vi "Main.vi"() -> ()   [LabVIEW 2015, in "Stock.lvlib"]
doc: "This template is based off of the Queued Message Handler design pattern and the Queued Message Handler project template that ships with LabVIEW.\n\nThe main difference is that the queue is private to this module and communication between modules is performed via Broadcast and Request events.\n\nRequest events are wrapped in public API methods and are handled in the Event Handling Loop (EHL) of this VI. Any module can register for Broadcast events sent by this module. The EHL generates messages based on user interface actions.\n\nThe Message Handling Loop (MHL) processes messages generated by the EHL, or by other messages. The messages are string values, so new messages can be added easily to the Message Cases case structure in the MHL. Each message cluster can also provide an optional value for Message Data, which is a variant that can be converted to whatever message-specific data is required.\n_____\nBased on Delacor QMH Project Template 4.2.1.64."
uses:
  Stock.lvlib
  <vilib>/Delacor/Delacor QMH/Libraries/Module Admin_class/Delacor_lib_QMH_Module Admin.lvclass
  Module Data--cluster.ctl
  Products.ctl
  <vilib>/Delacor/Delacor QMH/Libraries/Message Queue_class/Delacor_lib_QMH_Message Queue.lvclass/Delacor_lib_QMH_Message Queue.ctl
  Stop Argument--cluster.ctl
  <vilib>/Delacor/Delacor QMH/Libraries/Module Admin_class/Delacor_lib_QMH_Module Admin.lvclass/Delacor_lib_QMH_Module Admin.ctl
  In Stock and Price Argument--cluster.ctl
  In Stock and Price (Reply Payload)--cluster.ctl
  Reduce Stock Level Argument--cluster.ctl
  Reduce Stock Level (Reply Payload)--cluster.ctl
  <vilib>/Utility/miscctls.llb/LVPointTypeDef.ctl
  <vilib>/Delacor/Delacor QMH/Libraries/Message Queue_class/Delacor_lib_QMH_Enqueue Message (Single).vi
  <vilib>/Delacor/Delacor QMH/Libraries/Module Admin_class/Delacor_lib_QMH_Get External Launch.vi
  <vilib>/Utility/error.llb/Error Cluster From Error Code.vi
  <vilib>/ErrorRing/Error Ring.xnode
  <vilib>/Delacor/Delacor QMH/Libraries/Message Queue_class/Delacor_lib_QMH_Message Queue.lvclass
panel:
  out "Stock Levels":T1(array[cluster]) {"Price" format="£%.2f"; "Stock Level" scale=0.0..58.0}
  in  "Simulate MHL Error":bool
  in  "Simulate EHL Error":bool
  out "error out":errorcluster
  in  "Module Admin":refnum<class "Delacor_lib_QMH_Module Admin.lvclass">
  out "Status":string
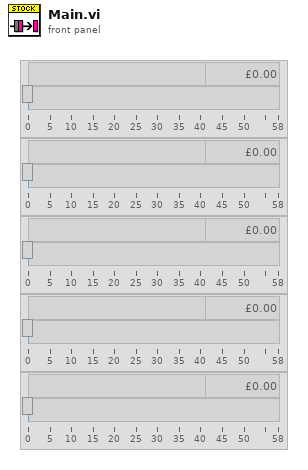
[diagram p1: front panel]
types:
  T1 = cluster{"Name":string, "Price":dbl, "Stock Level":dbl}[]
  T2 = typedef "Stock.lvlib/Request Events--cluster.ctl" = cluster{"Stop Module":refnum<user-event>, "Show Panel":refnum<user-event>, "Hide Panel":refnum<user-event>, "Get Module Execution Status":refnum<user-event>, "Show Diagram":refnum<user-event>, "In Stock and Price":refnum<user-event>, "Reduce Stock Level":refnum<user-event>}
  T3 = typedef "Stock.lvlib/Module Data--cluster.ctl" = cluster{"Status":string, "Stock":T4[], "Stock File Path":path}
  T4 = typedef "Stock.lvlib/Products.ctl" = cluster{"Name":string, "Price (pence/cents)":u32, "Stock Level":u32}
  T5 = enum32{"invalid lock state", "Not Locked", "Locked (No Password)", "Password-protected"}
  T6 = typedef "Stock.lvlib/Stop Argument--cluster.ctl" = cluster{"Origin":string, "Exit via Stop Module Req?":bool, "Wait for Module to stop?":bool}
  T7 = typedef "Stock.lvlib/In Stock and Price Argument--cluster.ctl" = cluster{"Stock Item":u32, "Wait Notifier":refnum<notifier>, "wait for reply":bool}
  T8 = typedef "Stock.lvlib/Reduce Stock Level Argument--cluster.ctl" = cluster{"Product":i32, "Wait Notifier":refnum<notifier>, "wait for reply":bool}
  T9 = typedef "LVPointTypeDef.ctl" = cluster{"Horizontal":i16, "Vertical":i16}
  T10 = typedef "Stock.lvlib/In Stock and Price (Reply Payload)--cluster.ctl" = cluster{"In Stock?":bool, "Price (Pence)":u32, "In Stock and Price_error":errorcluster}
  T11 = typedef "Stock.lvlib/Reduce Stock Level (Reply Payload)--cluster.ctl" = cluster{"Sucessful?":bool, "Reduce Stock Level_error":errorcluster}
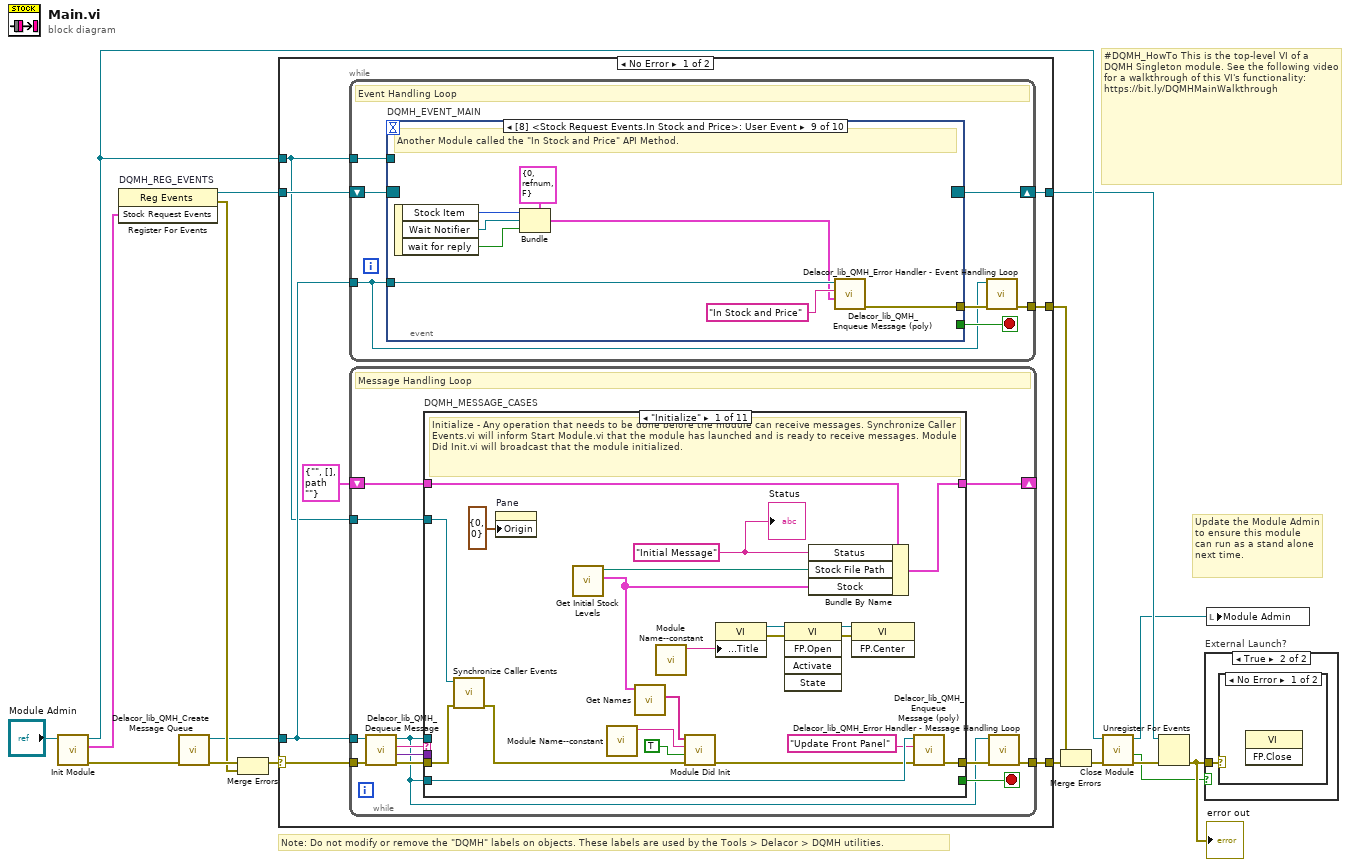
[diagram p0: block diagram]
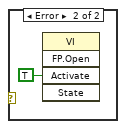
[diagram p3: hidden frame]
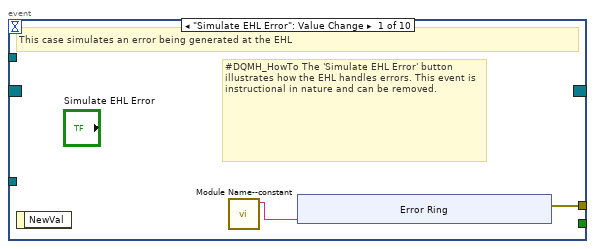
[diagram p4: hidden frame]
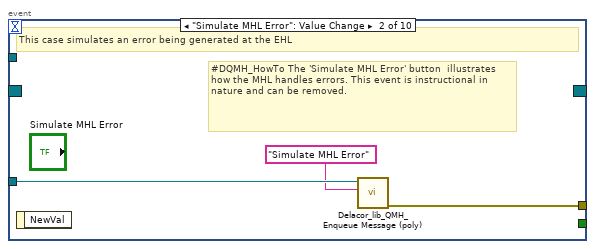
[diagram p5: hidden frame]
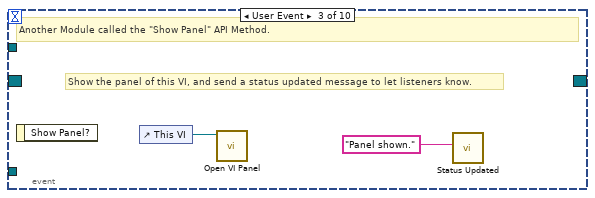
[diagram p6: hidden frame]
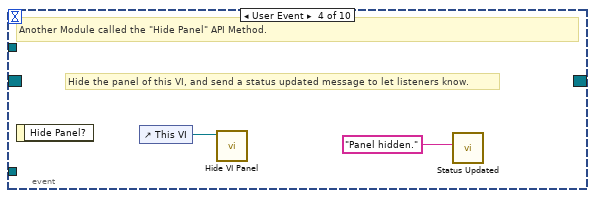
[diagram p7: hidden frame]
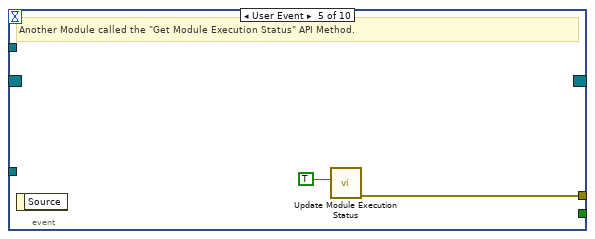
[diagram p8: hidden frame]
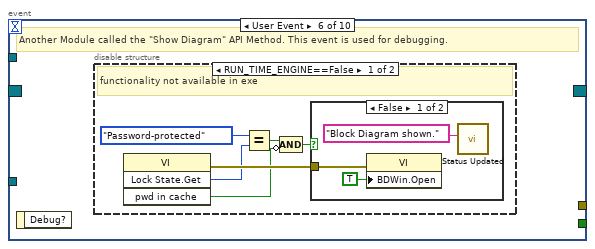
[diagram p9: hidden frame]
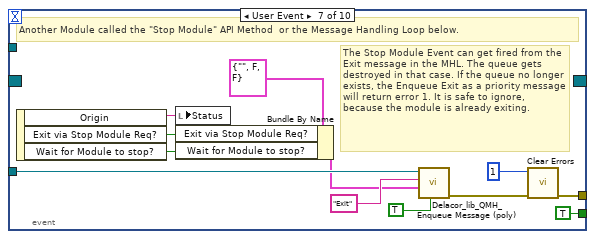
[diagram p12: hidden frame]
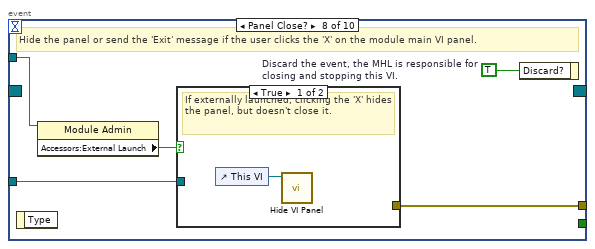
[diagram p13: hidden frame]
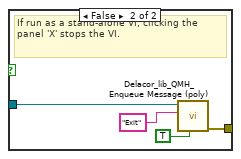
[diagram p14: hidden frame]
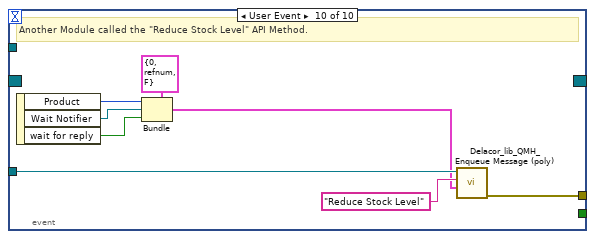
[diagram p15: hidden frame]
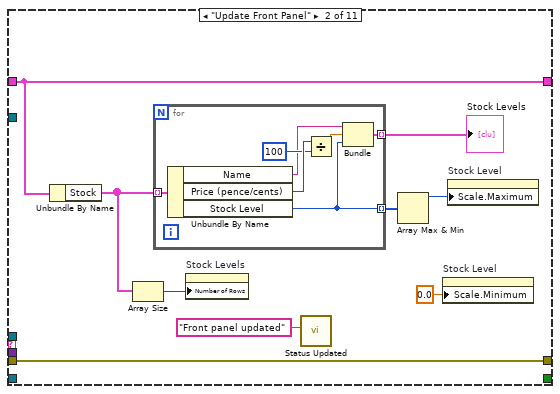
[diagram p16: hidden frame]
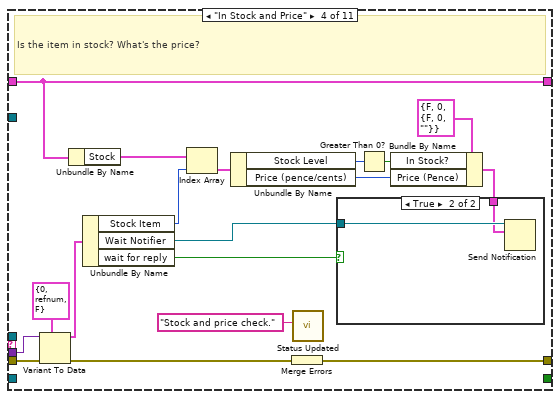
[diagram p18: hidden frame]
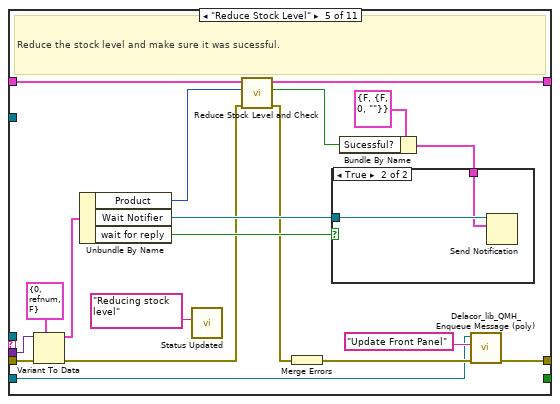
[diagram p20: hidden frame]
diagram:
  # "#DQMH_HowTo This is the top-level VI of a DQMH Singleton module. See the following video for a walkthrough of this VI's functionality: https://bit.ly/DQMHMainWalkthrough"
  # "Note: Do not modify or remove the \"DQMH\" labels on objects. These labels are used by the Tools > Delacor > DQMH utilities."
  # "Update the Module Admin to ensure this module can run as a stand alone next time."
  n1 = call "Init Module.vi"("Singleton Module Admin in"="Module Admin") -> ("error out"=w16:errorcluster, "Stock Request Events"=w5:T2, "Singleton Module Admin out"=w8:refnum<class "Delacor_lib_QMH_Module Admin.lvclass">)  [unwired: 8 in]
  n2 = register-events "DQMH_REG_EVENTS"(w5) -> (reference out=w6:refnum<event-registration>, error out=w9:errorcluster)  [unwired: 2 in]
  n3 = call <vilib>:"Delacor_lib_QMH_Create Message Queue.vi"("error in (no error)"=w16) -> ("error out"=w11:errorcluster, "Message Queue"=w4:refnum<class "Delacor_lib_QMH_Message Queue.lvclass">)  [unwired: 9 in]
  n4 = Merge Errors(w11, w9) -> (w10:errorcluster)
  n5 = case shown="No Error" w10 {
    selector: w10 -> [w23 w259]
    tunnel: [w25 w259] -> w17
    tunnel: [w22 w256] -> w7
    tunnel: w6 -> [w20 w256]
    tunnel: w4 -> [w19 _]
    tunnel: [w24 _] -> w14
    tunnel: w8 -> [w18 w252]
    frame No Error {
      n6 = while {
        tunnel: w19 -> [w26]
        shift-right: [w29] -> w22
        shift-left: w20 -> [w30]
        tunnel: [w31] -> w24
        tunnel: w18 -> [w27]
        stop <- w28 stop-if-true
        # "Event Handling Loop"
        n7 = event "DQMH_EVENT_MAIN" shown="[8] <Stock Request Events.In Stock and Price>: User Event" {
          selector: w30 -> [_ _ _ _ _ _ _ _ _ _]
          dyn-events: [_ _ _ _ _ _ _ _ _ _] -> w29
          timeout: _ -> [_ _ _ _ _ _ _ _ _ _]
          tunnel: [_ _ _ _ _ _ TRUE ("Discard?") _ _ _] -> w28
          tunnel: w26 -> [_ w43 _ _ _ _ w67 w74 w89 w97]
          tunnel: [w34 w44 _ _ w50 _ w70 w76 w82 w90] -> w32
          tunnel: w27 -> [_ _ _ _ _ _ _ w73 _ _]
          event "Simulate EHL Error": Value Change {
            # "#DQMH_HowTo The 'Simulate EHL Error' button  illustrates how the EHL handles errors. This event is instructional in nature and can be removed."
            # "This case simulates an error being generated at the EHL"
            n8 = event-data() -> ()  [unwired: 1 in, 1 out]
            n9 = call "Module Name--constant.vi"() -> ("Module Name"=w33:string)  [unwired: 11 in]
            n10 = xnode "Error Ring"("parameter 0"=w33) -> ("error out"=w34:errorcluster)
          }
          event "Simulate MHL Error": Value Change {
            # "#DQMH_HowTo The 'Simulate MHL Error' button  illustrates how the MHL handles errors. This event is instructional in nature and can be removed."
            # "This case simulates an error being generated at the EHL"
            n11 = event-data() -> ()  [unwired: 1 in, 1 out]
            n12 = call-poly <vilib>:"Delacor_lib_QMH_Enqueue Message (poly).vi"("Message"="Simulate MHL Error", "Message Queue in"=w43) -> ("error out"=w44:errorcluster)  [unwired: 8 in, 1 out]
          }
          event User Event {
            # "Show the panel of this VI, and send a status updated message to let listeners know."
            # "Another Module called the \"Show Panel\" API Method."
            n13 = event-data() -> ()  [unwired: 1 in, 1 out]
            n14 = control-ref of="This VI"() -> (w46:refnum<vi>)
            n15 = call "Open VI Panel.vi"("VI"=w46) -> ()  [unwired: 10 in, 1 out]
            n16 = call "Status Updated.vi"("Status"="Panel shown." ("format string")) -> ()  [unwired: 10 in, 1 out]
          }
          event User Event {
            # "Hide the panel of this VI, and send a status updated message to let listeners know."
            # "Another Module called the \"Hide Panel\" API Method."
            n17 = event-data() -> ()  [unwired: 1 in, 1 out]
            n18 = control-ref of="This VI"() -> (w48:refnum<vi>)
            n19 = call "Hide VI Panel.vi"("VI"=w48) -> ()  [unwired: 10 in, 1 out]
            n20 = call "Status Updated.vi"("Status"="Panel hidden." ("format string")) -> ()  [unwired: 10 in, 1 out]
          }
          event User Event {
            # "Another Module called the \"Get Module Execution Status\" API Method."
            n21 = event-data() -> ()  [unwired: 1 in, 1 out]
            n22 = call "Update Module Execution Status.vi"("Running?"=TRUE) -> ("error out"=w50:errorcluster)  [unwired: 10 in]
          }
          event User Event {
            # "Another Module called the \"Show Diagram\" API Method. This event is used for debugging."
            n23 = event-data() -> ()  [unwired: 1 in, 1 out]
            n24 = disable-structure shown="RUN_TIME_ENGINE==False" {
              frame condition #0 (active) {
                # "functionality not available in exe"
                n25 = invoke class="VI" method="Lock State.Get"() -> (error out=w56:errorcluster, "Get Lock State"=w55:T5, "pwd in cache"=w52:bool)  [unwired: 4 in, 1 out]
                n26 = Equal?(x=T5."Password-protected", y=w55) -> (x = y?=w53:bool)
                n27 = Compound Arithmetic op=AND(w53, invert w52) -> (w51:bool)
                n28 = case shown="False" w51 {
                  tunnel: w56 -> [w59 _]
                  frame False {
                    n29 = property class="VI"(error in=w59, "BDWin.Open"=TRUE ("Block Diagram Window:Open")) -> ()  [unwired: 1 in, 2 out]
                    n30 = call "Status Updated.vi"("Status"="Block Diagram shown." ("format string")) -> ()  [unwired: 10 in, 1 out]
                  }
                  frame True {
                    # "Password-protected VI, and the password is not in the cache. Do not show the diagram."
                  }
                }
              }
              frame condition #1 {
              }
            }
          }
          event User Event {
            # "The Stop Module Event can get fired from the Exit message in the MHL. The queue gets destroyed in that case. If the queue no longer exists, the Enqueue Exit as a priority message will return error 1. It is safe to ignore, because the module is already exiting."
            # "Another Module called the \"Stop Module\" API Method  or the Message Handling Loop below."
            n31 = event-data() -> ("Origin"=w66:string, "Exit via Stop Module Req?"=w62:bool, "Wait for Module to stop?"=w61:bool)  [unwired: 1 in]
            n32 = local write "Status"(w66) -> ()
            n33 = Bundle By Name(cluster=T6 {"Origin"="", "Exit via Stop Module Req?"=FALSE, "Wait for Module to stop?"=FALSE} ("Stop Argument"), "Exit via Stop Module Req?"=w62, "Wait for Module to stop?"=w61) -> (w60:T6)
            n34 = call-poly <vilib>:"Delacor_lib_QMH_Enqueue Message (poly).vi"("Priority Message? (F)"=TRUE, "Message Data"=w60, "Message"="Exit", "Message Queue in"=w67) -> ("error out"=w71:errorcluster)  [unwired: 6 in, 1 out]
            n35 = call <vilib>:"Clear Errors.vi"("error in (no error)"=w71, "specific error code to clear (0: all)"=1) -> ("error out"=w70:errorcluster)  [unwired: 4 in, 1 out]
          }
          event Panel Close? {
            w75 = TRUE  # Discard the event, the MHL is responsible for closing and stopping this VI.
            # "Hide the panel or send the 'Exit' message if the user clicks the 'X' on the module main VI panel."
            n36 = event-data() -> ()  [unwired: 1 in, 1 out]
            n37 = property class="Module Admin"(reference=w73) -> ("Accessors:External Launch"=w72:bool)  [unwired: 1 in, 2 out]
            n38 = case shown="True" w72 {
              tunnel: w74 -> [_ w80]
              tunnel: [_ w81] -> w76
              frame True {
                # "If externally launched, clicking the 'X' hides the panel, but doesn't close it."
                n39 = control-ref of="This VI"() -> (w77:refnum<vi>)
                n40 = call "Hide VI Panel.vi"("VI"=w77) -> ()  [unwired: 10 in, 1 out]
              }
              frame False {
                # "If run as a stand-alone VI, clicking the panel 'X' stops the VI."
                n41 = call-poly <vilib>:"Delacor_lib_QMH_Enqueue Message (poly).vi"("Priority Message? (F)"=TRUE, "Message"="Exit", "Message Queue in"=w80) -> ("error out"=w81:errorcluster)  [unwired: 7 in, 1 out]
              }
            }
            n42 = event-data("Discard?"=w75) -> ()  [unwired: 1 in, 1 out]
          }
          event User Event {
            # "Another Module called the \"In Stock and Price\" API Method."
            n43 = event-data() -> ("Stock Item"=w85:u32, "Wait Notifier"=w84:refnum<notifier>, "wait for reply"=w83:bool)  [unwired: 1 in]
            n44 = Bundle(cluster=T7 {"Stock Item"=0, "Wait Notifier"=refnum, "wait for reply"=FALSE} ("In Stock and Price Argument"), "Stock Item"=w85, "Wait Notifier"=w84, "wait for reply"=w83) -> (w86:T7)
            n45 = call-poly <vilib>:"Delacor_lib_QMH_Enqueue Message (poly).vi"("Message Data"=w86, "Message"="In Stock and Price", "Message Queue in"=w89) -> ("error out"=w82:errorcluster)  [unwired: 7 in, 1 out]
          }
          event User Event {
            # "Another Module called the \"Reduce Stock Level\" API Method."
            n46 = event-data() -> ("Product"=w93:i32, "Wait Notifier"=w92:refnum<notifier>, "wait for reply"=w91:bool)  [unwired: 1 in]
            n47 = Bundle(cluster=T8 {"Product"=0, "Wait Notifier"=refnum, "wait for reply"=FALSE} ("Reduce Stock Level Argument"), "Product"=w93, "Wait Notifier"=w92, "wait for reply"=w91) -> (w94:T8)
            n48 = call-poly <vilib>:"Delacor_lib_QMH_Enqueue Message (poly).vi"("Message Data"=w94, "Message"="Reduce Stock Level", "Message Queue in"=w97) -> ("error out"=w90:errorcluster)  [unwired: 7 in, 1 out]
          }
        }
        n49 = call-dynamic "Delacor_lib_QMH_Error Handler - Event Handling Loop.vi"("error in (no error)"=w32, "Message Queue in"=w26) -> ("dup error in"=w31:errorcluster)  [unwired: 8 in, 1 out]
      }
      n50 = while {
        tunnel: w19 -> [w100]
        shift-right: [w104] -> _
        shift-left: T3 {"Status"="", "Stock"=[], "Stock File Path"=path ""} ("Data Cluster") -> [w105]
        tunnel: w23 -> [w108]
        tunnel: [w106] -> w25
        tunnel: w18 -> [w99]
        stop <- w103 stop-if-true
        # "Message Handling Loop"
        n51 = call-dynamic "Delacor_lib_QMH_Dequeue Message.vi"("error in (no error)"=w108, "Message Queue in"=w100) -> ("error out"=w107:errorcluster, "Message Data"=w101:variant, "Message"=w102:string, "Message Queue out"=w98:refnum<class "Delacor_lib_QMH_Message Queue.lvclass">)  [unwired: 6 in]
        n52 = case "DQMH_MESSAGE_CASES" shown="\"Initialize\"" w102 {
          selector: w102 -> [_ _ _ _ _ _ _ _ _ _ w239]
          tunnel: w98 -> [_ _ _ _ _ _ _ _ w209 w231 _]
          tunnel: w107 -> [w130 w139 w148 w166 w187 w192 w194 w199 w216 w237 w241]
          tunnel: [w118 w139 w148 w157 w171 w191 w194 w198 w212 w234 w242] -> w109
          tunnel: w105 -> [w127 w138 w147 w156 w179 w190 w193 w196 w211 w230 w240]
          tunnel: [w126 w138 w147 w156 w178 w190 w193 w196 w211 w230 w240] -> w104
          tunnel: [_ _ _ _ _ _ _ _ _ w229 _] -> w103
          tunnel: w101 -> [_ _ _ w164 w186 _ _ _ w210 w228 _]
          tunnel: w99 -> [w128 _ _ _ _ _ _ _ w208 w223 _]
          tunnel: w98 -> [w121 _ _ _ w170 _ _ _ _ _ _]
          frame "Initialize" {
            w122 = "Initial Message" ("Initial Message")
            # "Initialize - Any operation that needs to be done before the module can receive messages. Synchronize Caller Events.vi will inform Start Module.vi that the module has launched and is ready to receive messages. Module Did Init.vi will broadcast that the module initialized."
            n53 = call "Synchronize Caller Events.vi"("error in (no error)"=w130, "Singleton Module Admin in"=w128) -> ("error out"=w129:errorcluster)  [unwired: 8 in, 1 out]
            n54 = property on="Pane" class="Pane"("Origin"=T9 {"Horizontal"=0, "Vertical"=0}) -> ()  [unwired: 2 in, 2 out]
            n55 = call "Get Initial Stock Levels.vi"() -> ("Stock"=w115:T4[], "Stock file path"=w114:path)  [unwired: 10 in]
            n56 = call "Module Name--constant.vi"() -> ("Module Name"=w124:string)  [unwired: 11 in]
            n57 = call "Get Names.vi"("Stock"=w115) -> ("Product Names"=w117:string[])  [unwired: 10 in]
            n58 = call "Module Name--constant.vi"() -> ("Module Name"=w116:string)  [unwired: 11 in]
            n59 = call "Module Did Init.vi"("error in (no error)"=w129, "Initialized?"=TRUE, "Origin"=w124, "Product Names"=w117) -> ("error out"=w119:errorcluster)  [unwired: 7 in]
            n60 = property class="VI"("Front Panel.Title"=w116) -> (reference out=w111:refnum<vi>, error out=w110:errorcluster)  [unwired: 2 in]
            n61 = invoke class="VI" method="FP.Open"(reference=w111, error in=w110) -> (reference out=w112:refnum<vi>, error out=w113:errorcluster)  [unwired: 3 in, 3 out]
            n62 = Bundle By Name(cluster=w127, "Status"=w122, "Stock File Path"=w114, "Stock"=w115) -> (w126:T3)
            n63 = invoke class="VI" method="FP.Center"(reference=w112, error in=w113) -> ()  [unwired: 1 in, 3 out]
            n64 = call-poly <vilib>:"Delacor_lib_QMH_Enqueue Message (poly).vi"("error in (no error)"=w119, "Message"="Update Front Panel" ("Initial Message"), "Message Queue in"=w121) -> ("error out"=w118:errorcluster)  [unwired: 7 in, 1 out]
            "Status" <- w122
          }
          frame "Update Front Panel" {
            n65 = Unbundle By Name(w138) -> ("Stock"=w134:T4[])
            n66 = Array Size(array=w134) -> (size(s)=w133:i32)
            n67 = for {
              tunnel: w134 -> [w146] mode=indexing
              tunnel: [w143] -> w136 mode=indexing
              tunnel: [w140] -> w137 mode=indexing
              n68 = Unbundle By Name(w146) -> ("Name"=w141:string, "Price (pence/cents)"=w145:u32, "Stock Level"=w143:u32)
              n69 = Divide(x=w145, y=u32 100) -> (x/y=w142:dbl)
              n70 = Bundle("Name"=w141, w142, "Stock Level"=w143) -> (w140:cluster{"Name":string, dbl, "Stock Level":u32})  [unwired: 1 in]
            }
            "Stock Levels" <- w137
            n71 = property on="Stock Levels" class="Arr (strict)"("Number of Rows"=w133) -> ()  [unwired: 2 in, 2 out]
            n72 = call "Status Updated.vi"("Status"="Front panel updated") -> ()  [unwired: 10 in, 1 out]
            n73 = Array Max & Min(array=w136) -> (max value=w135:u32)  [unwired: 3 out]
            n74 = property on="Stock Level" class="Slide (strict)"("Scale.Minimum"=0.0 ("Scale.Range:Minimum")) -> ()  [unwired: 2 in, 2 out]
            n75 = property on="Stock Level" class="Slide (strict)"("Scale.Maximum"=w135) -> ()  [unwired: 2 in, 2 out]
          }
          frame "--- Module Specific ---" {
            # "Separator -- The following cases handle messages specific to this Module."
          }
          frame "In Stock and Price" {
            # "Is the item in stock? What's the price?"
            n76 = Variant To Data(error in=w166, type=T7 {"Stock Item"=0, "Wait Notifier"=refnum, "wait for reply"=FALSE} ("In Stock and Price Argument"), Variant=w164) -> (data=w162:T7, error out=w165:errorcluster)
            n77 = Unbundle By Name(w156) -> ("Stock"=w155:T4[])
            n78 = Unbundle By Name(w162) -> ("Stock Item"=w154:u32, "Wait Notifier"=w161:refnum<notifier>, "wait for reply"=w160:bool)
            n79 = Index Array(array=w155, index=w154) -> (element=w153:T4)
            n80 = Unbundle By Name(w153) -> ("Stock Level"=w151:u32, "Price (pence/cents)"=w152:u32)
            n81 = Merge Errors(w165) -> (w157:errorcluster)
            n82 = call "Status Updated.vi"("Status"="Stock and price check.") -> ()  [unwired: 10 in, 1 out]
            n83 = Greater Than 0?(x=w151) -> (x > 0?=w150:bool)
            n84 = Bundle By Name(cluster=T10 {"In Stock?"=FALSE, "Price (Pence)"=0, "In Stock and Price_error"={"status"=FALSE, "code"=0, "source"=""}} ("In Stock and Price (Reply Payload)"), "In Stock?"=w150, "Price (Pence)"=w152) -> (w159:T10)
            n85 = case shown="True" w160 {
              tunnel: w161 -> [_ w168]
              tunnel: w159 -> [_ w167]
              frame False {
              }
              frame True {
                n86 = Send Notification(notification=w167, notifier=w168) -> ()  [unwired: 1 in, 2 out]
              }
            }
          }
          frame "Reduce Stock Level" {
            # "Reduce the stock level and make sure it was sucessful."
            n87 = Variant To Data(error in=w187, type=T8 {"Product"=0, "Wait Notifier"=refnum, "wait for reply"=FALSE} ("Reduce Stock Level Argument"), Variant=w186) -> (data=w184:T8, error out=w175:errorcluster)
            n88 = Unbundle By Name(w184) -> ("Product"=w177:i32, "Wait Notifier"=w183:refnum<notifier>, "wait for reply"=w182:bool)
            n89 = call "Status Updated.vi"("Status"="Reducing stock level") -> ()  [unwired: 10 in, 1 out]
            n90 = call "Reduce Stock Level and Check.vi"("error in (no error)"=w175, "Product Index"=w177, "Data Cluster"=w179) -> ("error out"=w174:errorcluster, "Sucessful"=w176:bool, "Data Cluster Out"=w178:T3)  [unwired: 6 in]
            n91 = Merge Errors(w174) -> (w172:errorcluster)
            n92 = Bundle By Name(cluster=T11 {"Sucessful?"=FALSE, "Reduce Stock Level_error"={"status"=FALSE, "code"=0, "source"=""}} ("Reduce Stock Level (Reply Payload)"), "Sucessful?"=w176) -> (w181:T11)
            n93 = case shown="True" w182 {
              tunnel: w183 -> [_ w189]
              tunnel: w181 -> [_ w188]
              frame False {
              }
              frame True {
                n94 = Send Notification(notification=w188, notifier=w189) -> ()  [unwired: 1 in, 2 out]
              }
            }
            n95 = call-poly <vilib>:"Delacor_lib_QMH_Enqueue Message (poly).vi"("error in (no error)"=w172, "Message"="Update Front Panel" ("Initial Message"), "Message Queue in"=w170) -> ("error out"=w171:errorcluster)  [unwired: 7 in, 1 out]
          }
          frame "---Copy This Frame---" {
            # "Duplicate this frame when creating new messages.  Change this comment in the duplicated frame to describe this message."
            n96 = Merge Errors(w192) -> (w191:errorcluster)
          }
          frame "--- Exit and Error Handling---" {
            # "Separator - The following cases handle errors and exit messages."
          }
          frame "Simulate MHL Error" {
            # "#DQMH_HowTo The 'Simulate MHL Error' button  illustrates how the MHL handles errors. This event is instructional in nature and can be removed."
            # "Simulate an error occurring at the MHL"
            n97 = call "Module Name--constant.vi"() -> ("Module Name"=w195:string)  [unwired: 11 in]
            n98 = xnode "Error Ring"("parameter 0"=w195) -> ("error out"=w197:errorcluster)
            n99 = Merge Errors(w199, w197) -> (w198:errorcluster)
          }
          frame "Error" {
            # "#CodeRecommended - If you ever change the name of this \"Error\" message, you'll need to update the name in the Check Loop Error.vi as well."
            # "#CodeRecommended - If the module is running in standalone mode (External Launch = FALSE), this code will pop up an error dialog and call the 'Exit' message if an error occurs. Add more fine-grained error handling here."
            # "Error - Check the error message data and respond accordingly. This message is sent by the \"Error Handler\" VIs at the end of each loop in this application."
            n100 = property class="Module Admin"(reference=w208) -> ("Accessors:External Launch"=w207:bool)  [unwired: 1 in, 2 out]
            n101 = Variant To Data(error in=w216, type=errorcluster {"status"=FALSE, "code"=0, "source"=""} ("error constant"), Variant=w210) -> (data=w217:errorcluster, error out=w214:errorcluster)
            n102 = call "Error Reported.vi"("Error"=w217) -> ()  [unwired: 10 in, 1 out]
            n103 = case shown="True" w207 {
              tunnel: [w222 _] -> w213
              tunnel: w209 -> [w220 _]
              tunnel: w217 -> [w221 _]
              frame False {
                # "If the module is running standalone, then pop up an error dialog and call the \"Exit\" message."
                n104 = call <vilib>:"Simple Error Handler.vi"("error in (no error)"=w221) -> ()  [unwired: 4 in, 5 out]
                n105 = call-poly <vilib>:"Delacor_lib_QMH_Enqueue Message (poly).vi"("Priority Message? (F)"=TRUE, "Message"="Exit", "Message Queue in"=w220) -> ("error out"=w222:errorcluster)  [unwired: 7 in, 1 out]
              }
              frame True {
                # "If the module was launched externally, calling the Error Reported broadcast VI is the only action performed by the \"Error\" message. The module's caller can then process the error appropriately."
              }
            }
            n106 = Merge Errors(w214, w213) -> (w212:errorcluster)
            n107 = local write "error out"(w212) -> ()
          }
          frame "Exit" {
            w227 = 91  # 91: not all Exit messages will have an argument
            w229 = TRUE  # Stop the VI
            # "Release the message queue reference"
            # "#CodeNeeded - Add any required cleanup code here"
            # "Exit - Exit the application."
            n108 = Variant To Data(error in=w237, type=T6 {"Origin"="", "Exit via Stop Module Req?"=FALSE, "Wait for Module to stop?"=FALSE} ("Stop Argument"), Variant=w228) -> (data=w225:T6, error out=w233:errorcluster)
            n109 = call <vilib>:"Clear Errors.vi"("error in (no error)"=w233, "specific error code to clear (0: all)"=w227) -> ("error out"=w236:errorcluster)  [unwired: 4 in, 1 out]
            n110 = control-ref of="This VI"() -> (w224:refnum<vi>)
            n111 = call-dynamic "Delacor_lib_QMH_Release Message Queue.vi"("error in (no error)"=w236, "Message Queue"=w231) -> ("error out"=w235:errorcluster)  [unwired: 9 in]
            n112 = call "Handle Exit.vi"("Stop Argument"=w225, "Admin in"=w223, "VI reference"=w224) -> ("error out"=w232:errorcluster)  [unwired: 7 in, 1 out]
            n113 = Merge Errors(w235, w232) -> (w234:errorcluster)
          }
          frame Default {
            # "'Default' case only runs if there is a message that isn't defined in any of the other cases.  Output a programming error."
            n114 = call "Module Name--constant.vi"() -> ("Module Name"=w238:string)  [unwired: 11 in]
            n115 = xnode "Error Ring"("parameter 0"=w239, "parameter 1"=w238) -> ("error out"=w243:errorcluster)
            n116 = Merge Errors(w241, w243) -> (w242:errorcluster)
          }
        }
        n117 = call-dynamic "Delacor_lib_QMH_Error Handler - Message Handling Loop.vi"("error in (no error)"=w109, "Message Queue in"=w98) -> ("dup error in"=w106:errorcluster)  [unwired: 8 in, 1 out]
      }
    }
    frame Error {
      # "Synchronize Caller Events.vi will inform Start Module.vi that the module has launched and will let the code calling Start Module.vi register for broadcasts and would permit the caller receive the broadcast that an error occurred at launch time."
      n118 = call "Synchronize Caller Events.vi"("Singleton Module Admin in"=w252) -> ("error out"=w257:errorcluster)  [unwired: 9 in, 1 out]
      n119 = call "Module Name--constant.vi"() -> ("Module Name"=w255:string)  [unwired: 11 in]
      n120 = Format Into String(format string="An error occurred during initialization. %s is no longer running.", w255) -> (resulting string=w253:string)  [unwired: 2 in, 1 out]
      n121 = Merge Errors(w259, w257) -> (w258:errorcluster)
      n122 = call "Error Reported.vi"("Additional Information"=w253, "Error"=w258) -> ()  [unwired: 9 in, 1 out]
    }
  }
  n123 = Merge Errors(w14, w17) -> (w13:errorcluster)
  n124 = call "Close Module.vi"("error in (no error)"=w13, "Module Admin in"=w8) -> ("error out"=w15:errorcluster, "External Launch"=w1:bool, "Module Admin out"=w2:refnum<class "Delacor_lib_QMH_Module Admin.lvclass">)  [unwired: 7 in]
  n125 = Unregister For Events(event registration refnum=w7, error in=w15) -> (error out=w12:errorcluster)
  "error out" <- w12
  n126 = case "External Launch?" shown="True" w1 {
    tunnel: w12 -> [_ w260]
    frame False {
    }
    frame True {
      n127 = case shown="No Error" w260 {
        frame No Error {
          n128 = invoke class="VI" method="FP.Close"() -> ()  [unwired: 3 in, 3 out]
        }
        frame Error {
          n129 = invoke class="VI" method="FP.Open"("Activate"=TRUE ("Activate?")) -> ()  [unwired: 4 in, 5 out]
        }
      }
    }
  }
  n130 = local write "Module Admin"(w2) -> ()
